vi "from string.vi"(8 "error in":errorcluster, 9 "data":string, 10 "version":string, 11 "configuration in":refnum<class "channel configuration.lvclass">) -> (0 "error out":errorcluster, 3 "configuration out":refnum<class "channel configuration.lvclass">)   [LabVIEW 2013, in "channel configuration.lvclass"]
doc: "Provides an interface for loading a module configuration from a file or other serialized data source. It is recommended that all children of this class store data in two sets--data required for its own initialization, and any data required for parent initialization--and that each implementation uses the <b>Call Parent Method</b> primitive to de-serialize parent information."
uses:
  channel configuration.lvclass
  ChannelData.ctl
  Configuration Framework/serializable configuration/NISE_CEF_serializable configuration.lvclass
  channel configuration.lvclass/channel configuration.ctl
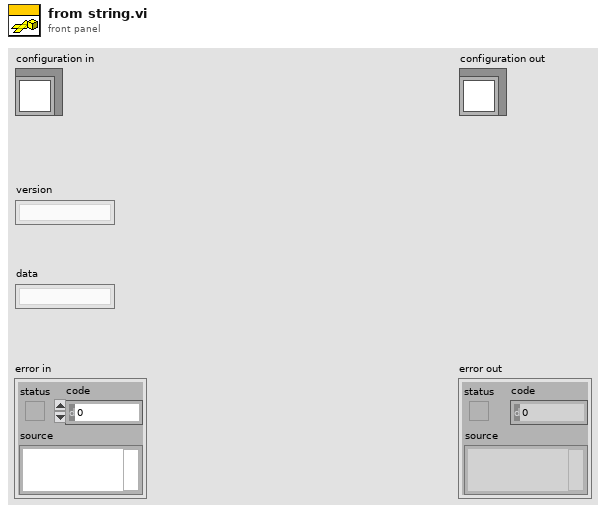
[diagram p1: front panel]
types:
  T1 = typedef "channel configuration.lvclass/ChannelData.ctl" = cluster{"channel group":string, "channel name":string, "IO":string, "sensor ID":string, "description":string, "system":string, "channel type":string}
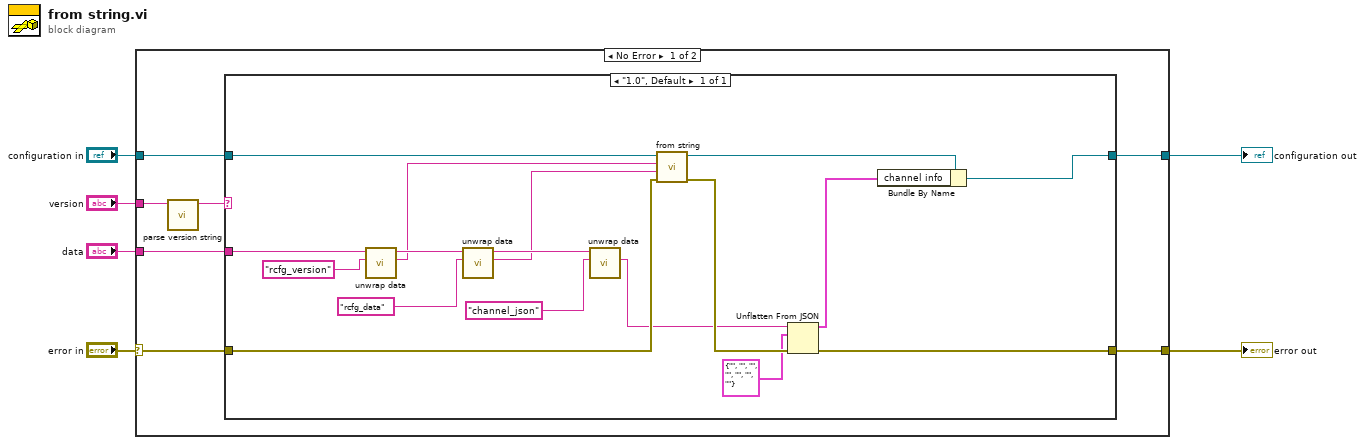
[diagram p0: block diagram]
diagram:
  n1 = case shown="No Error" "error in" {
    selector: "error in" -> [w8 w32]
    tunnel: "data" -> [w13 _]
    tunnel: "configuration in" -> [w12 w31]
    tunnel: [w11 w31] -> w4
    tunnel: [w7 w32] -> w5
    tunnel: "version" -> [w10 _]
    frame No Error {
      n2 = call "parse version string.vi"("full version"=w10) -> ("major.minor version"=w9:string)  [unwired: 7 in, 3 out]
      n3 = case shown="\"1.0\", Default" w9 {
        tunnel: w13 -> [w30]
        tunnel: w8 -> [w26]
        tunnel: w12 -> [w24]
        tunnel: [w22] -> w11
        tunnel: [w21] -> w7
        frame "1.0", Default {
          n4 = call "unwrap data.vi"("identifier"="rcfg_version" ("additional identifier"), "data to unwrap"=w30) -> ("unwrapped data"=w14:string, "remaining string"=w28:string)  [unwired: 8 in]
          n5 = call "unwrap data.vi"("identifier"="rcfg_data" ("additional identifier"), "data to unwrap"=w28) -> ("unwrapped data"=w15:string, "remaining string"=w18:string)  [unwired: 8 in]
          n6 = call "unwrap data.vi"("identifier"="channel_json" ("additional identifier"), "data to unwrap"=w18) -> ("unwrapped data"=w17:string)  [unwired: 8 in, 1 out]
          n7 = call-parent "from string.vi"("error in"=w26, "data"=w15, "version"=w14, "configuration in"=w24) -> ("error out"=w25:errorcluster, "configuration out"=w23:refnum<class "channel configuration.lvclass">)  [unwired: 6 in]
          n8 = Unflatten From JSON(JSON string=w17, type and defaults=T1 {"channel group"="", "channel name"="", "IO"="", "sensor ID"="", "description"="", "system"="", "channel type"=""} ("channel info"), error in (no error)=w25) -> (value=w19:T1, error out=w21:errorcluster)  [unwired: 4 in]
          n9 = Bundle By Name(cluster=w23, "channel info"=w19) -> (w22:refnum<class "channel configuration.lvclass">)
        }
      }
    }
    frame Error {
    }
  }
  "error out" <- w5
  "configuration out" <- w4
